vi "replaceQueryTokens.vi"(8 "error in (no error)":errorcluster, 10 "Query In":string, 11 "BankingTransaction in":refnum<class "BankingTransaction.lvclass">) -> (0 "error out":errorcluster, 2 "Query Out":string, 3 "BankingTransaction out":refnum<class "BankingTransaction.lvclass">)   [LabVIEW 2020, in "BankingTransaction.lvclass"]
uses:
  BankingTransaction.lvclass
  BankingTransaction.lvclass/BankingTransaction.ctl
  Transaction/Transaction.lvclass
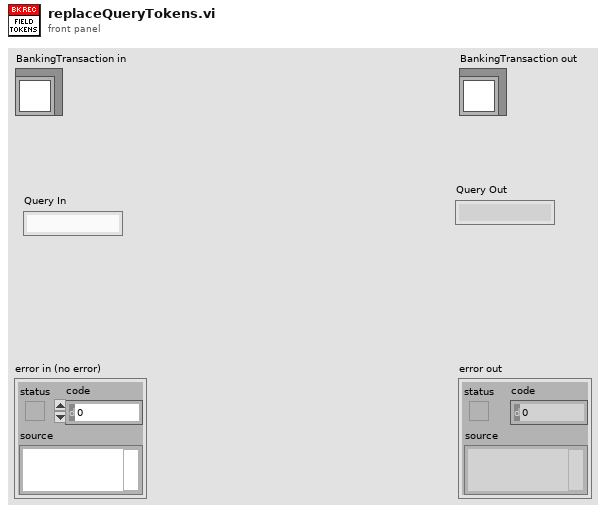
[diagram p1: front panel]
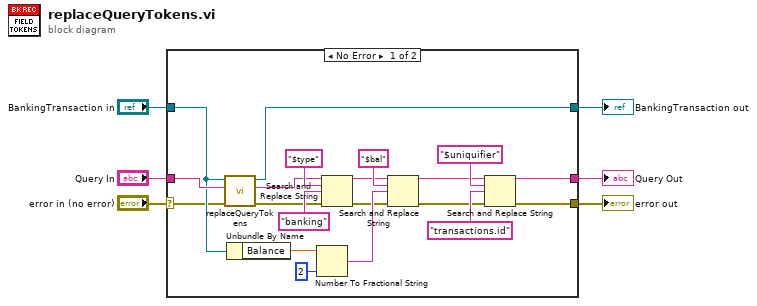
[diagram p0: block diagram]
diagram:
  n1 = case shown="No Error" "error in (no error)" {
    selector: "error in (no error)" -> [w13 w28]
    tunnel: [w26 w29] -> w6
    tunnel: "Query In" -> [w25 w27]
    tunnel: "BankingTransaction in" -> [w16 w29]
    tunnel: [w7 w28] -> w3
    tunnel: [w8 w27] -> w2
    frame No Error {
      n2 = call-parent "replaceQueryTokens.vi"("error in (no error)"=w13, "Query In"=w25, "Transaction in"=w16) -> ("error out"=w21:errorcluster, "Query Out"=w22:string, "Transaction out"=w26:refnum<class "BankingTransaction.lvclass">)  [unwired: 6 in]
      n3 = Unbundle By Name(w16) -> ("Balance"=w19:dbl)
      n4 = Number To Fractional String(number=w19, precision (6)=i16 2) -> (F-format string=w18:string)  [unwired: 2 in]
      n5 = Search and Replace String(input string=w22, search string="$type", replace string="banking" ("replace string (\"\")"), error in=w21) -> (result string=w15:string, error out=w14:errorcluster)  [unwired: 4 in, 2 out]
      n6 = Search and Replace String(input string=w15, search string="$bal", replace string=w18, error in=w14) -> (result string=w10:string, error out=w9:errorcluster)  [unwired: 4 in, 2 out]
      n7 = Search and Replace String(input string=w10, search string="$uniquifier", replace string="transactions.id", error in=w9) -> (result string=w8:string, error out=w7:errorcluster)  [unwired: 4 in, 2 out]
    }
    frame Error {
    }
  }
  "error out" <- w3
  "BankingTransaction out" <- w6
  "Query Out" <- w2
